vi "info_test.vi"() -> ()   [LabVIEW 2013]
panel:
  in  "String":string
  in  "btn exit":bool
  out "error out":errorcluster
  in  "Value":string
  in  "btn add stuff":bool
  out "text ref":refnum<vi>
  in  "btn view":bool
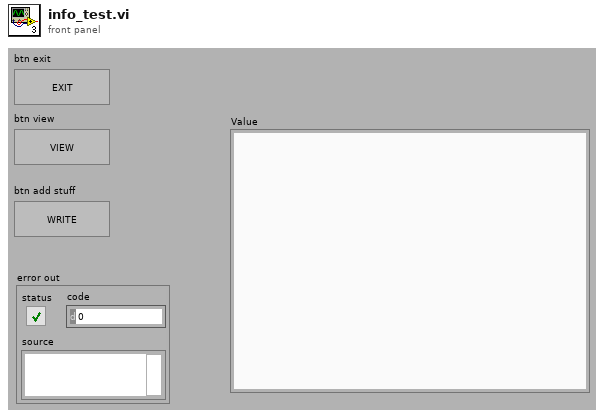
[diagram p1: front panel]
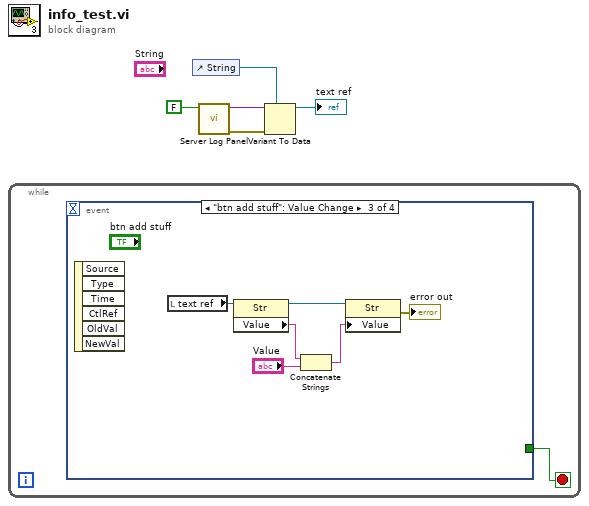
[diagram p0: block diagram]
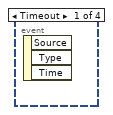
[diagram p2: hidden frame]
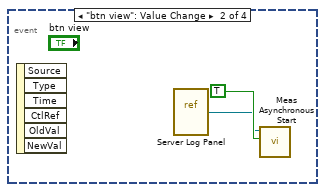
[diagram p3: hidden frame]
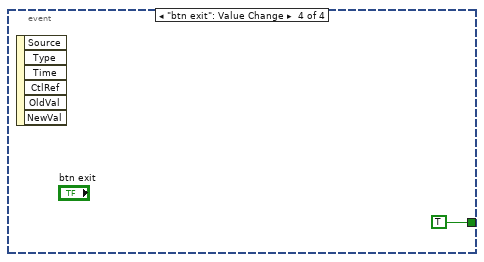
[diagram p4: hidden frame]
diagram:
  n1 = while {
    stop <- w6 stop-if-true
    n2 = event shown="[2] \"btn add stuff\": Value Change" {
      selector: _ -> [_ _ _ _]
      dyn-events: _ -> [_ _ _ _]
      timeout: _ -> [_ _ _ _]
      tunnel: [_ _ _ TRUE] -> w6
      event Timeout {
        n3 = event-data() -> ()  [unwired: 1 in, 3 out]
      }
      event "btn view": Value Change {
        n4 = event-data() -> ()  [unwired: 1 in, 6 out]
        n5 = vi-ref "Server Log Panel.vi"() -> (w7:refnum<vi>)
        n6 = call "Meas Asynchronous Start.vi"("parameter in"=TRUE, "Static VI reference in (empty)"=w7) -> ()  [unwired: 8 in, 2 out]
      }
      event "btn add stuff": Value Change {
        n7 = event-data() -> ()  [unwired: 1 in, 6 out]
        n8 = local read "text ref"() -> (w12:refnum<vi>)
        n9 = property class="Str"(reference=w12) -> (reference out=w13:refnum<vi>, "Value"=w11:string)  [unwired: 1 in, 1 out]
        n10 = Concatenate Strings(w11, "Value") -> (w10:string)
        n11 = property class="Str"(reference=w13, "Value"=w10) -> (error out=→"error out":errorcluster)  [unwired: 1 in, 1 out]
      }
      event "btn exit": Value Change {
        n12 = event-data() -> ()  [unwired: 1 in, 6 out]
      }
    }
  }
  n13 = control-ref of="String"() -> (w2:refnum<vi>)
  n14 = call "Server Log Panel.vi"("open window (false)"=FALSE) -> ("error out"=w5:errorcluster, "text ref"=w4:variant)  [unwired: 9 in]
  n15 = Variant To Data(error in=w5, type=w2, Variant=w4) -> (data=→"text ref":refnum<vi>)  [unwired: 1 out]
